vi "Configuration Error Message - Text--Const.vi"() -> (1 "Button Text":string="Error!", 2 "User Message":string="Error.\n\nThe minimum current limit must be less than the maximum current limit.\nThe maximum current limit must be less than the maximum current.")   [LabVIEW 2017, in "DTacq Plot Display Library.lvlib"]
doc: "A string containing an error message for the user;\n\nThe minimum current limit must be less than the maximum current limit.\nThe maximum current limit must be less than the maximum current."
uses:
  DTacq Plot Display Library.lvlib
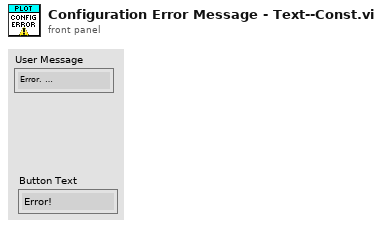
[diagram p1: front panel]
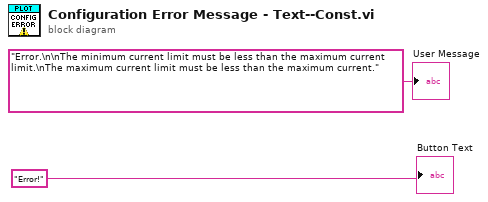
[diagram p0: block diagram]
diagram:
  "User Message" <- "Error.\n\nThe minimum current limit must be less than the maximum current limit.\nThe maximum current limit must be less than the maximum current."
  "Button Text" <- "Error!"
